vi "Test Tilt & LED.vi"() -> ()   [LabVIEW 2015]
uses:
  Controls/Led Control.ctl
  <vilib>/Analysis/baseanly.llb/Mean (DBL).vi
  <vilib>/myRIO/Common/Instrument Driver Framework/myRIO v1.0/UART/vis/myRIO v1.0 Close UART.vi
  <vilib>/myRIO/Common/Instrument Driver Framework/Utilities/vis/FPGA Ref Manager.vi
  <vilib>/myRIO/Common/Instrument Driver Framework/myRIO v1.0/myRIO v1.0 Reset FPGA.vi
  <vilib>/myRIO/Common/Instrument Driver Framework/myRIO v1.0/IRQ/vis/myRIO v1.0 IRQ Info FGV.vi
  <vilib>/myRIO/Common/Instrument Driver Framework/myRIO v1.0/IRQ/vis/myRIO v1.0 Timer IRQ Info FGV.vi
  <vilib>/myRIO/Common/Instrument Driver Framework/myRIO v1.0/IRQ/vis/myRIO v1.0 ISR Agent.vi
  <vilib>/myRIO/Instrument Drivers/Utilities/Utilities.lvlib
  <vilib>/Analysis/NI_AALBase.lvlib
panel:
  in  "Led Option x":T1
  in  "Set LED":bool
  in  "Set Tilt":bool
  in  "tilt degree x":i32=12
  out "mean":dbl format="%0.2f"
  out "period":u32
  out "error out":errorcluster
  in  "Led Option 0":T1=enum."LED_RED"
  in  "tilt degree 0":i32=12
  in  "Depth Format":T2(ring)=enum."FREENECT_DEPTH_10BIT"
  in  "stop":bool
  out "Depth":T3(plugin-control)
  # "0-23"
  # "Low--->8,6 ms\nTiny--->2,5 ms"
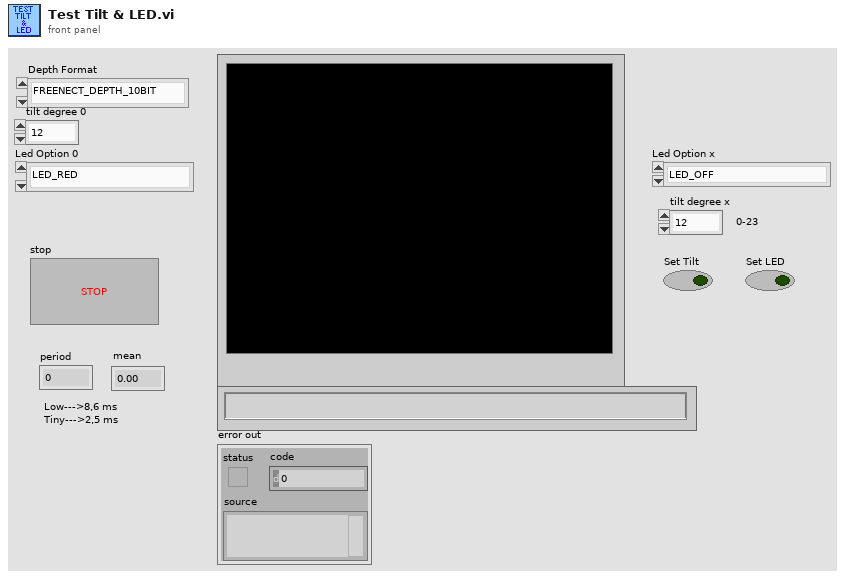
[diagram p1: front panel]
types:
  T1 = typedef "Led Control.ctl" = enum32{"LED_OFF", "LED_GREEN", "LED_RED", "LED_YELLOW", "LED_BLINK_GREEN", "LED_BLINK_GREEN2", "LED_BLINK_RED_YELLOW"}
  T2 = enum32{"FREENECT_DEPTH_11BIT", "FREENECT_DEPTH_10BIT", "FREENECT_DEPTH_11BIT_PACKED", "FREENECT_DEPTH_10BIT_PACKED", "FREENECT_DEPTH_REGISTERED", "FREENECT_DEPTH_MM"}
  T3 = typedef "IMAQ Image.ctl" = refnum<image>
  T4 = typedef "Image Type" = u32
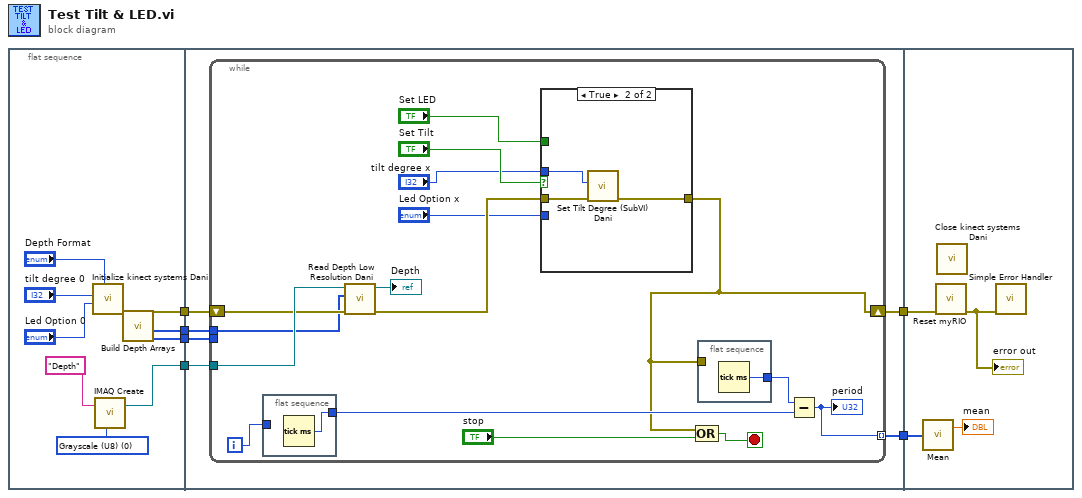
[diagram p0: block diagram]
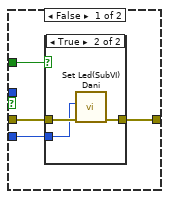
[diagram p2: hidden frame]
diagram:
  n1 = flat-sequence {
    tunnel: [w15] -> w6
    tunnel: [w14] -> w4
    tunnel: [w8] -> w3
    tunnel: [w7] -> w2
    tunnel: w6 -> [w21]
    tunnel: [w20] -> w5
    tunnel: w4 -> [w19]
    tunnel: w3 -> [w18]
    tunnel: w2 -> [w17]
    tunnel: [w16] -> w1
    tunnel: w5 -> [w54]
    tunnel: w1 -> [w52]
    frame #0 {
      w9 = T4 0 items=["Grayscale (U8)", "Grayscale (I16)", "Grayscale (SGL)", "Complex (CSG)", "RGB (U32)", "HSL (U32)", "RGB (U64)", "Grayscale (U16)"] ("Image Type")
      n2 = call "Initialize kinect systems Dani.vi"("Depth Format"="Depth Format", "Led Option"="Led Option 0", "tilt degree"="tilt degree 0") -> ("error out"=w15:errorcluster)  [unwired: 8 in]
      n3 = call "IMAQ Create"("Image Name"="Depth", "Image Type"=w9) -> ("New Image"=w14:T3)  [unwired: 3 in, 1 out]
      n4 = call "Build Depth Arrays.vi"() -> ("Array Tiny"=w7:u16[], "Array Low"=w8:u16[])  [unwired: 10 in]
    }
    frame #1 {
      n5 = while {
        shift-right: [w22] -> w20
        shift-left: w21 -> [w30]
        tunnel: w19 -> [w31]
        tunnel: w18 -> [w29]
        tunnel: w17 -> [_]
        tunnel: [w32] -> w16 mode=indexing
        i -> [w35]
        stop <- w36 stop-if-true
        n6 = flat-sequence {
          tunnel: w35 -> [_]
          tunnel: [w50] -> w33
          frame #0 {
            n7 = Tick Count (ms)() -> (millisecond timer value=w50:u32)
          }
        }
        n8 = call "Read Depth Low Resolution Dani.vi"("error in (no error)"=w30, "depth"=w29, "Image In"=w31) -> ("error out"=w27:errorcluster, "Image Out"=→"Depth":T3)  [unwired: 7 in]
        n9 = case shown="True" "Set Tilt" {
          tunnel: [w41 w48] -> w22
          tunnel: w27 -> [w40 w46]
          tunnel: "Set LED" -> [w39 _]
          tunnel: "Led Option x" -> [w38 _]
          tunnel: "tilt degree x" -> [_ w47]
          frame False {
            n10 = case shown="True" w39 {
              tunnel: [w42 w45] -> w41
              tunnel: w40 -> [w42 w44]
              tunnel: w38 -> [_ w43]
              frame False {
              }
              frame True {
                n11 = call "Set Led(SubVI) Dani.vi"("error in (no error)"=w44, "Led Option"=w43) -> ("error out"=w45:errorcluster)  [unwired: 9 in]
              }
            }
          }
          frame True {
            n12 = call "Set Tilt Degree (SubVI) Dani.vi"("degree"=w47, "error in (no error)"=w46) -> ("error out"=w48:errorcluster)  [unwired: 8 in]
          }
        }
        n13 = Compound Arithmetic op=OR(w22, "stop") -> (w36:bool)
        n14 = flat-sequence {
          tunnel: [w49] -> w34
          tunnel: w22 -> [_]
          frame #0 {
            n15 = Tick Count (ms)() -> (millisecond timer value=w49:u32)
          }
        }
        n16 = Subtract(x=w34, y=w33) -> (x-y=w32:u32)
        "period" <- w32
      }
    }
    frame #2 {
      n17 = call-poly <vilib>:"Mean.vi"("X"=w52) -> ("mean"=→"mean":dbl)  [unwired: 1 out]
      n18 = call <vilib>:"Reset myRIO.vi"("error in (no error)"=w54) -> ("error out"=w53:errorcluster)  [unwired: 10 in]
      "error out" <- w53
      n19 = call "Close kinect systems Dani.vi"() -> ()  [unwired: 11 in, 1 out]
      n20 = call <vilib>:"Simple Error Handler.vi"("error in (no error)"=w53) -> ()  [unwired: 4 in, 5 out]
    }
  }
